vi "Populate Device Settings.vi"(8 "error in":errorcluster, 11 "UI Actor in":refnum<class "UI Actor.lvclass">) -> (0 "error out":errorcluster)   [LabVIEW 2019, in "UI Actor.lvlib" / "UI Actor.lvclass"]
uses:
  UI Actor.lvclass
  UI Actor.lvclass/UI Actor.ctl
  Controls/Device Settings.ctl
  UI Actor.lvlib
  Electronic Datasheet/Electronic Datasheet.lvclass
  <vilib>/Utility/Data Type/NI_Data Type.lvlib
  Core/Device Info/Device Info.lvclass
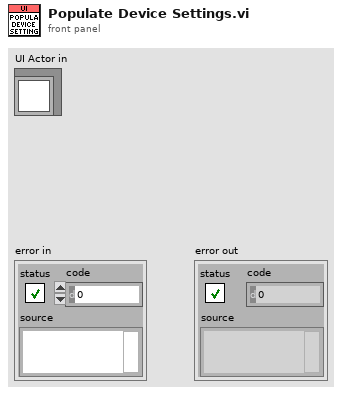
[diagram p1: front panel]
types:
  T1 = typedef "UI Actor.lvlib/Device Settings.ctl" = cluster{"SimpleBootUpSlave":bool, "SimpleBootUpMaster":bool}
  T2 = map{path, refnum<class "Electronic Datasheet.lvclass">}
  T3 = cluster{"VendorName":string, "VendorNumber":u32, "ProductName":string, "ProductNumber":u32, "RevisionNumber":u32, "OrderCode":string, "BaudRate_10":bool, "BaudRate_20":bool, "BaudRate_50":bool, "BaudRate_125":bool, "BaudRate_250":bool, "BaudRate_500":bool, "BaudRate_800":bool, "BaudRate_1000":bool, "BaudRate_auto":bool, "SimpleBootUpMaster":bool, "SimpleBootUpSlave":bool, "Granularity":u8, "DynamicChannelsSupported":bool, "CompactPDO":u8, "GroupMessaging":bool, "NrOfRXPDO":u16, "NrOfTXPDO":u16, "LSS_Supported":bool, "LSS_Master":bool, "NG_Slave":bool, "NG_Master":bool, "NrOfNG_MonitoredNodes":u16}
  T4 = enum16{"SimpleBootUpSlave", "SimpleBootUpMaster"}
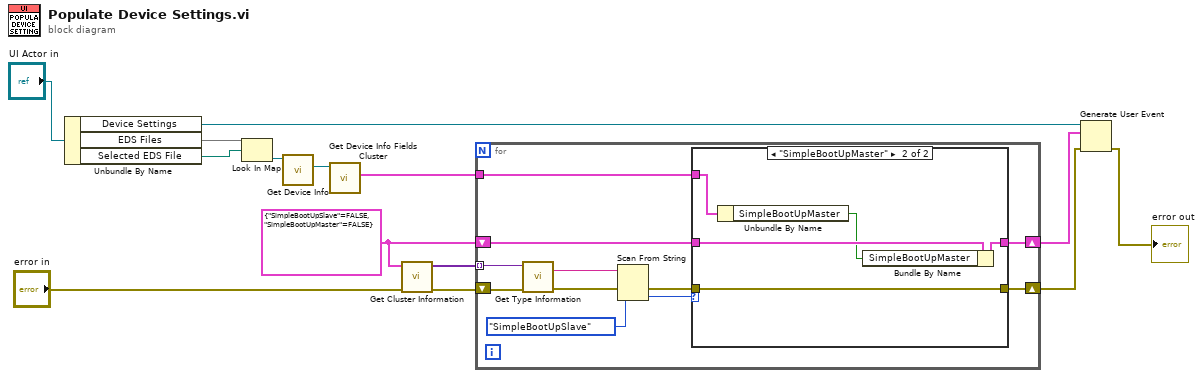
[diagram p0: block diagram]
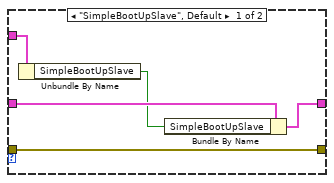
[diagram p2: hidden frame]
diagram:
  w3 = T1 {"SimpleBootUpSlave"=FALSE, "SimpleBootUpMaster"=FALSE} ("Device Settings")
  n1 = Unbundle By Name("UI Actor in") -> ("Device Settings"=w13:refnum<user-event>, "EDS Files"=w11:T2, "Selected EDS File"=w10:path)
  n2 = Look In Map(map=w11, key=w10) -> (value=w9:refnum<class "Electronic Datasheet.lvclass">)  [unwired: 1 in, 1 out]
  n3 = call "Get Device Info.vi"("reference in"=w9) -> ("Device Info"=w8:refnum<class "Device Info.lvclass">)  [unwired: 8 in, 2 out]
  n4 = call "Get Device Info Fields Cluster.vi"("Device Info in"=w8) -> ("Device Info"=w4:T3)  [unwired: 9 in, 1 out]
  n5 = call <vilib>:"Get Cluster Information.vi"("error in (no error)"="error in", "variant"=w3) -> ("error out"=w5:errorcluster, "cluster elements"=w7:variant[])  [unwired: 8 in]
  n6 = for {
    tunnel: w7 -> [w25] mode=indexing
    tunnel: w4 -> [w18]
    shift-right: [w17] -> w2
    shift-left: w3 -> [w19]
    shift-right: [w15] -> w1
    shift-left: w5 -> [w24]
    n7 = call <vilib>:"Get Type Information.vi"("error in (no error)"=w24, "variant"=w25) -> ("error out"=w22:errorcluster, "name"=w21:string)  [unwired: 5 in, 3 out]
    n8 = Scan From String(input string=w21, error in=w22, default 1=T4."SimpleBootUpSlave") -> (error out=w16:errorcluster, output 1=w20:T4)  [unwired: 2 in, 2 out]
    n9 = case shown="\"SimpleBootUpMaster\"" w20 {
      tunnel: w19 -> [w30 w34]
      tunnel: w18 -> [w29 w33]
      tunnel: [w27 w32] -> w17
      tunnel: w16 -> [w26 w35]
      tunnel: [w26 w35] -> w15
      frame "SimpleBootUpSlave", Default {
        n10 = Unbundle By Name(w29) -> ("SimpleBootUpSlave"=w28:bool)
        n11 = Bundle By Name(cluster=w30, "SimpleBootUpSlave"=w28) -> (w27:T1)
      }
      frame "SimpleBootUpMaster" {
        n12 = Unbundle By Name(w33) -> ("SimpleBootUpMaster"=w31:bool)
        n13 = Bundle By Name(cluster=w34, "SimpleBootUpMaster"=w31) -> (w32:T1)
      }
    }
  }
  n14 = Generate User Event(user event=w13, event data cluster=w2, error in=w1) -> (error out=→"error out":errorcluster)  [unwired: 1 in, 1 out]
